vi "Transmittance.vi"(1 "P1 Power":dbl[](array[numeric]), 2 "P1 Wavelength":dbl[](array[numeric]), 3 "P0 Power":dbl[](array[numeric]), 4 "P0 Wavelength":dbl[](array[numeric])) -> (0 "Transmittance":dbl[](array[numeric]))   [LabVIEW 2019]
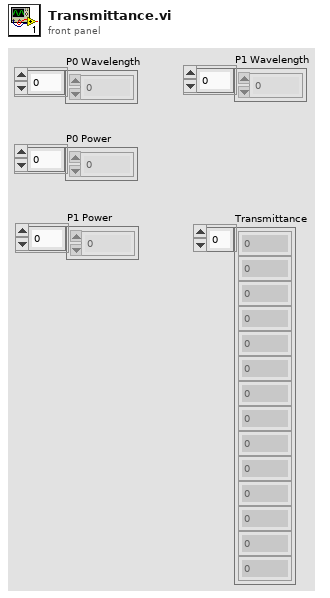
[diagram p1: front panel]
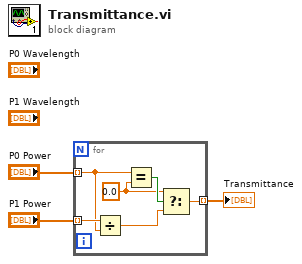
[diagram p0: block diagram]
diagram:
  n1 = for {
    tunnel: "P0 Power" -> [w8] mode=indexing
    tunnel: "P1 Power" -> [w9] mode=indexing
    tunnel: [w5] -> w1 mode=indexing
    w4 = 0.0 ("t")
    n2 = Divide(x=w9, y=w8) -> (x/y=w6:dbl)
    n3 = Equal?(x=w8, y=w4) -> (x = y?=w7:bool)
    n4 = Select(t=w4, s=w7, f=w6) -> (s? t:f=w5:dbl)
  }
  "Transmittance" <- w1
